vi "ExVar.vi"() -> ()   [LabVIEW 2018]
panel:
  out "n3":dbl
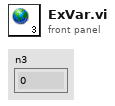
[diagram p1: front panel]
diagram:
